vi "Init Example Device.vi"(10 "Number of Channels":u32=1, 11 "ExampleDevice.lvclass":refnum<class "ExampleDevice.lvclass">) -> (3 "ExampleDevice.lvclass 2":refnum<class "ExampleDevice.lvclass">)   [LabVIEW 2023, in "ExampleDevice.lvclass"]
uses:
  ExampleDevice.lvclass
  ExampleDevice.lvclass/ExampleDevice.ctl
  Current Setpoint/Current Setpoint.lvclass
  Voltage Setpoint/Voltage Setpoint.lvclass
panel:
  out "Array 2":string[](array[string])
  out "Array":string[](array[string])
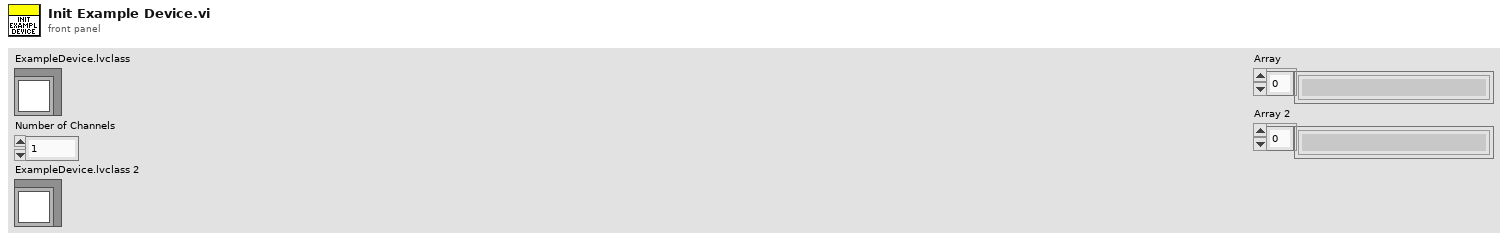
[diagram p1: front panel]
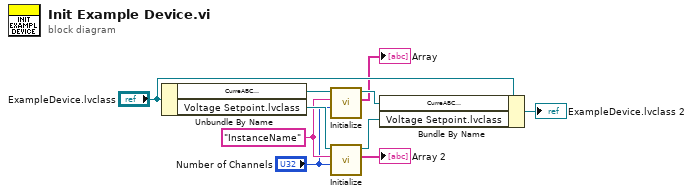
[diagram p0: block diagram]
diagram:
  w8 = "InstanceName" ("Plugin Name")
  n1 = Unbundle By Name("ExampleDevice.lvclass") -> ("CurreABC\n.lvclass"=w10:refnum<class "Current Setpoint.lvclass">, "Voltage Setpoint.lvclass"=w9:refnum<class "Voltage Setpoint.lvclass">)
  n2 = call-dynamic "Initialize.vi"("Number of Channels"="Number of Channels", "Plugin Name"=w8, "Current Setpoint in"=w10) -> ("Array"=→"Array":string[], "Current Setpoint out"=w5:refnum<class "Current Setpoint.lvclass">)  [unwired: 6 in, 1 out]
  n3 = call-dynamic "Initialize.vi"("Number of Channels"="Number of Channels", "Plugin Name"=w8, "Voltage Setpoint in"=w9) -> ("Array"=→"Array 2":string[], "Voltage Setpoint out"=w4:refnum<class "Voltage Setpoint.lvclass">)  [unwired: 6 in, 1 out]
  n4 = Bundle By Name(cluster="ExampleDevice.lvclass", "CurreABC\n.lvclass"=w5, "Voltage Setpoint.lvclass"=w4) -> (→"ExampleDevice.lvclass 2":refnum<class "ExampleDevice.lvclass">)
